vi "resonant.image queue to disk and to display queue_rrMD.vi"() -> ()   [LabVIEW 2012]
doc: "SciScan 1.0 151216"
uses:
  <vilib>/Utility/VariantDataType/Type.ctl
  Custom Controls/file format type def.ctl
  GFG/GFGnumericGet.vi
  GFG/GFGfpRefGet.vi
  GFG/GFGbooleanGet.vi
  image & display/save images/save channels to raw bin files.vi
  image & display/save images/save channels to interleaved multi-tiff files.vi
  image & display/save images/save channels to separate multi-tiff files.vi
  image & display/save images/save channels to stacked multi-tiff files.vi
  image & display/save images/save channels to interleaved tiff series.vi
  image & display/save images/save channels to separate tiff series.vi
  image & display/save images/save channels to stacked tiff series.vi
  GFG/GFG library.lvlib
  <vilib>/Utility/VariantDataType/VariantType.lvlib
panel:
  in  "Stop Button":bool
  out "VI is running":bool
  out "size(s)":i32[](array[numeric])
  out "error out 5":errorcluster
  out "error out 4":errorcluster
  out "error out 3":errorcluster
  out "error out 2":errorcluster
  out "# elements in image data queue":i32
  out "error out":errorcluster
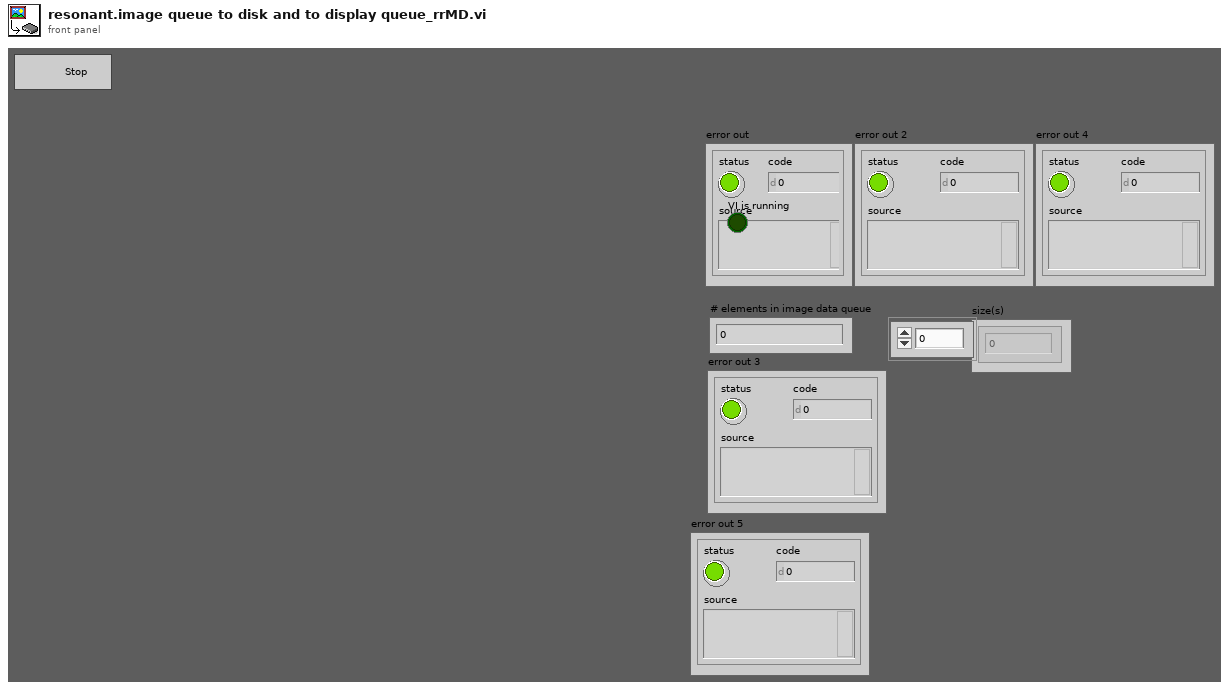
[diagram p1: front panel]
types:
  T1 = cluster{"Variable Name in":string, "Variant Out":variant}
  T2 = typedef "file format type def.ctl" = enum16{"16bit raw", "32bit raw", "16bit multi-tiff (interleave)", "16bit multi-tiff (separate)", "16bit multi-tiff (stacked)", "32bit multi-tiff (interleave)", "32bit multi-tiff (separate)", "32bit multi-tiff (stacked)", "16bit tiff series (interleave)", "16bit tiff series (separate)", "16bit tiff series (stacked)", "32bit tiff series (interleave)", "32bit tiff series (separate)", "32bit tiff series (stacked)"}
  T3 = enum8{"Enabled", "Disabled", "Disabled and Grayed Out"}
  T4 = cluster{"WaveformChartRef":refnum<vi>, "DigitalRef":refnum<vi>, "ArrayRef":refnum<vi>, "TabControlRef":refnum<vi>, "EnumRef":refnum<vi>, "RingRef":refnum<vi>, "BooleanRef":refnum<vi>, "KnobRef":refnum<vi>, "SlideRef":refnum<vi>, "PathRef":refnum<vi>, "StringRef":refnum<vi>, "ComboBox":refnum<vi>, "WaveformGraphRef":refnum<vi>}
  T5 = cluster{"NewVal":bool, "Event Registration Refnum":refnum<event-registration>}
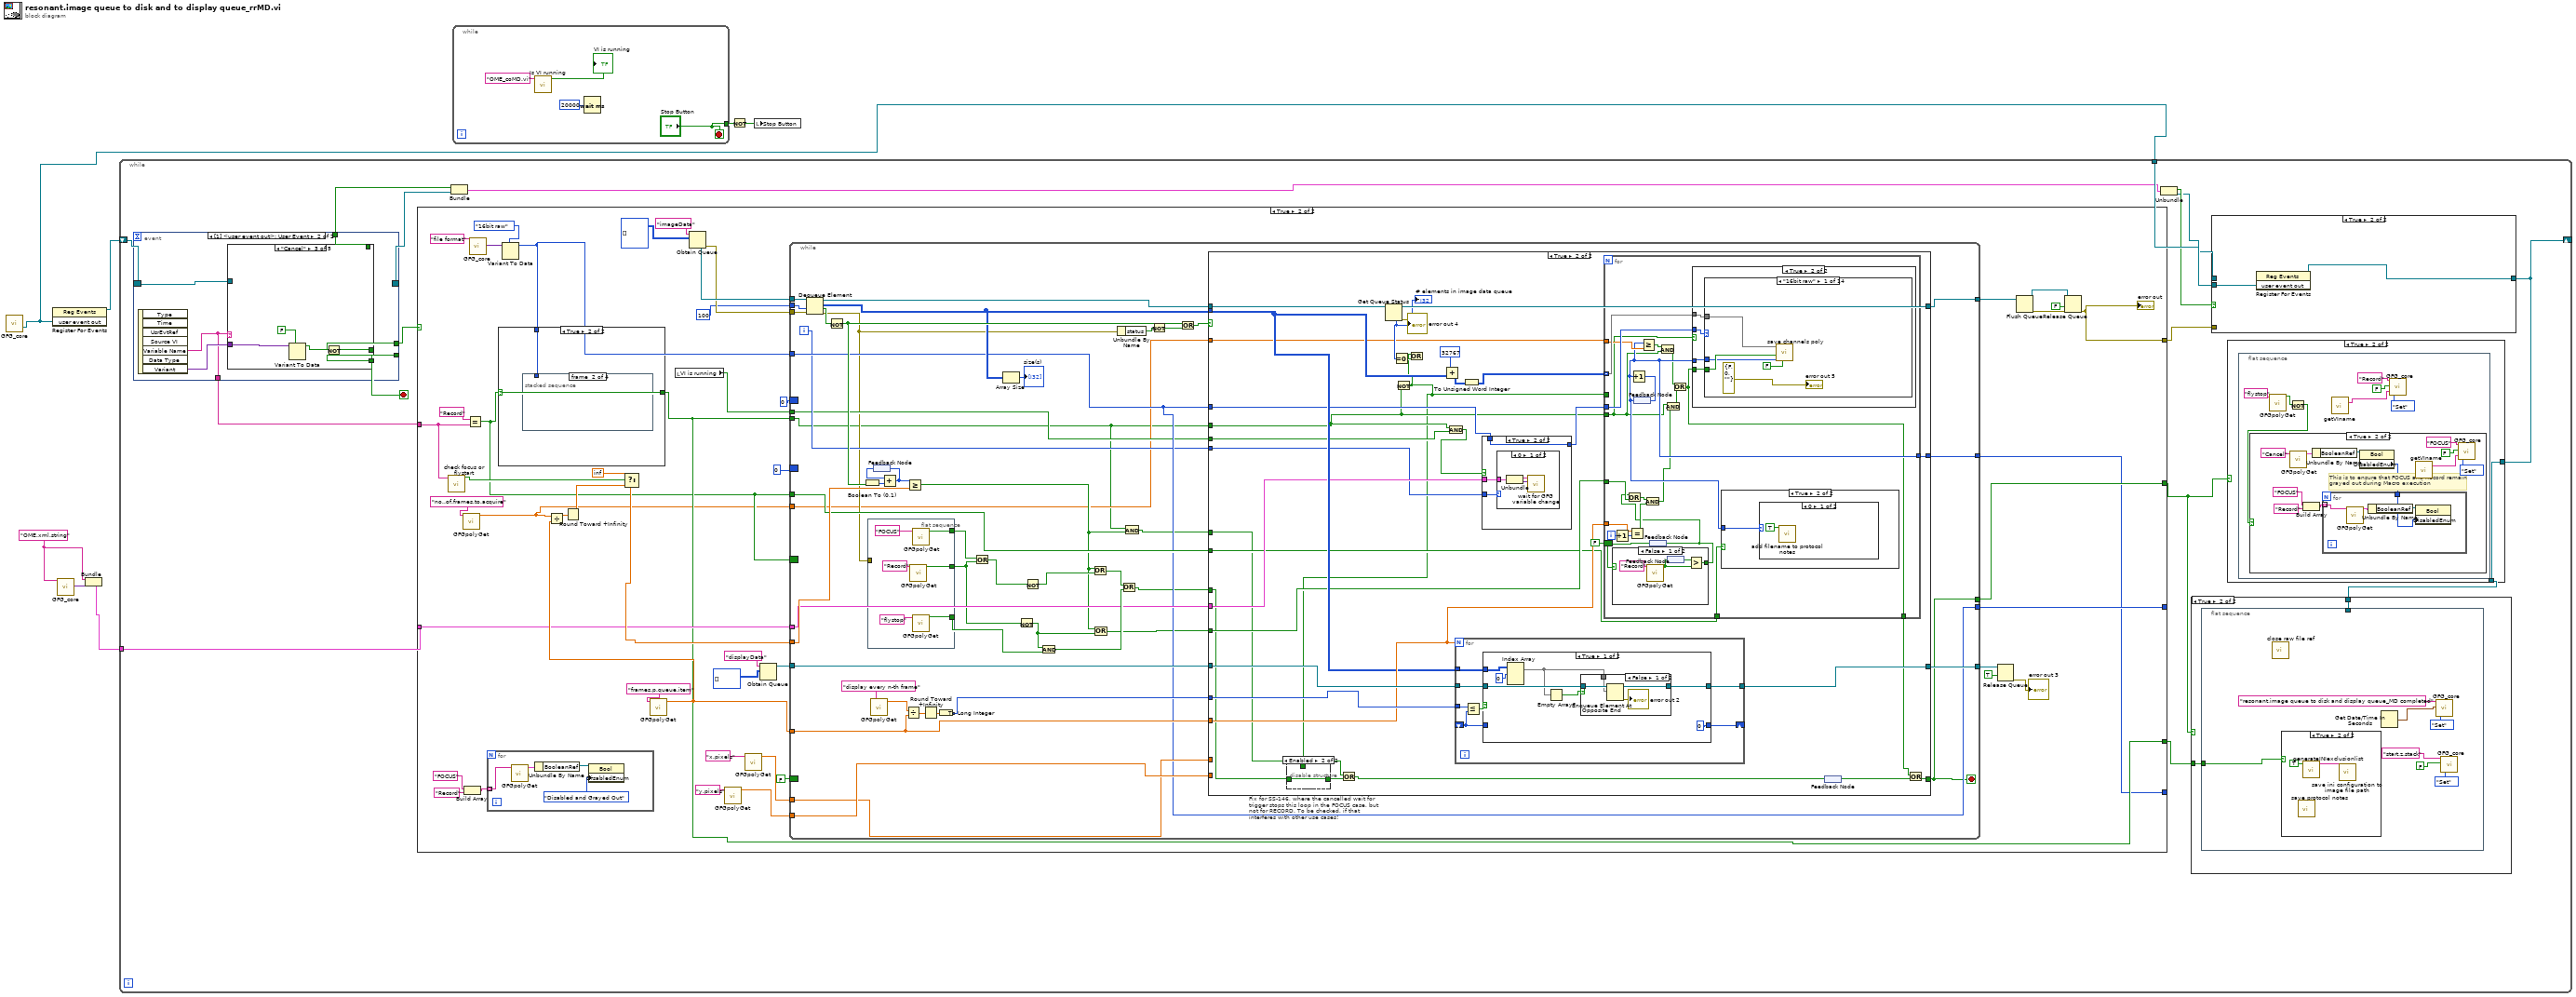
[diagram p0: block diagram]
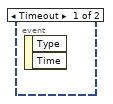
[diagram p7: hidden frame]
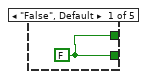
[diagram p8: hidden frame]
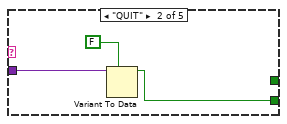
[diagram p9: hidden frame]
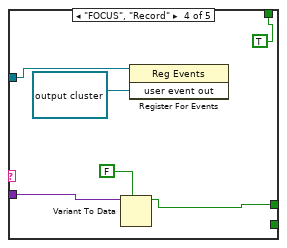
[diagram p10: hidden frame]
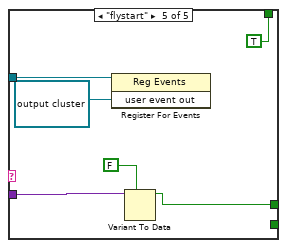
[diagram p11: hidden frame]
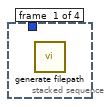
[diagram p14: hidden frame]
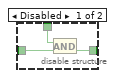
[diagram p18: hidden frame]
diagram:
  w4 = "OME.xml.string" ("Variable Name in")
  n1 = call "GFG_core.vi"() -> ("user event out"=w6:refnum<user-event>)  [unwired: 13 in, 6 out]
  n2 = register-events(w6) -> (reference out=w7:refnum<event-registration>)  [unwired: 2 in, 1 out]
  n3 = call "GFG_core.vi"("Variable Name in"=w4) -> ("Variant Out"=w5:variant)  [unwired: 12 in, 6 out]
  n4 = Bundle("Variable Name in"=w4, "Variant Out"=w5) -> (w3:T1)  [unwired: 1 in]
  n5 = while {
    shift-right: [w10] -> _
    shift-left: w7 -> [w20]
    tunnel: w6 -> [w19]
    tunnel: w3 -> [w12]
    stop <- w22 stop-if-true
    n6 = event shown="[1] <user event out>: User Event" {
      selector: w20 -> [_ w63]
      dyn-events: [_ _] -> w16
      timeout: _ -> [_ _]
      tunnel: [_ w67] -> w23
      tunnel: [_ w66] -> w22
      tunnel: [_ w64] -> w21
      tunnel: [_ w62] -> w17
      event Timeout {
        n7 = event-data() -> ()  [unwired: 1 in, 2 out]
      }
      event User Event {
        n8 = event-data() -> ("Variable Name"=w64:string, "Variant"=w65:variant)  [unwired: 1 in, 5 out]
        n9 = case shown="\"Cancel\"" w64 {
          tunnel: [w68 _ w72 w79 w85] -> w67
          tunnel: [w68 w69 _ _ _] -> w66
          tunnel: w65 -> [_ w71 w74 w80 w86]
          tunnel: w63 -> [_ _ _ w77 w83]
          tunnel: [_ _ _ TRUE ("NewVal") TRUE ("NewVal")] -> w62
          frame "False", Default {
            w68 = FALSE ("NewVal")
          }
          frame "QUIT" {
            n10 = Variant To Data(type=FALSE ("NewVal"), Variant=w71) -> (data=w69:bool)  [unwired: 1 in, 1 out]
          }
          frame "Cancel" {
            n11 = Variant To Data(type=FALSE ("NewVal"), Variant=w74) -> (data=w73:bool)  [unwired: 1 in, 1 out]
            n12 = Not(x=w73) -> (.not. x?=w72:bool)
          }
          frame "FOCUS", "Record" {
            n13 = Variant To Data(type=FALSE ("NewVal"), Variant=w80) -> (data=w79:bool)  [unwired: 1 in, 1 out]
            n14 = register-events(reference=w77, refnum<user-event> refnum ("user event out")) -> ()  [unwired: 1 in, 2 out]
          }
          frame "flystart" {
            n15 = register-events(reference=w83, refnum<user-event> refnum ("user event out")) -> ()  [unwired: 1 in, 2 out]
            n16 = Variant To Data(type=FALSE ("NewVal"), Variant=w86) -> (data=w85:bool)  [unwired: 1 in, 1 out]
          }
        }
      }
    }
    n17 = case shown="True" w23 {
      tunnel: w21 -> [_ w111]
      tunnel: [_ w120] -> w18
      tunnel: [_ w107] -> w8
      tunnel: w12 -> [_ w98]
      tunnel: [_ w97] -> w11
      tunnel: [_ w96] -> _
      tunnel: [_ w94] -> _
      frame False {
      }
      frame True {
        n18 = call "check focus or flystart.vi"("GFG variable name"=w111) -> ("Focus or flystart?"=w110:bool)  [unwired: 10 in]
        n19 = call-poly "GFGpolyGet.vi"("Variable Name in"="no..of.frames.to.acquire" ("Tag in")) -> ("Numeric"=w90:dbl)  [unwired: 8 in, 2 out]
        n20 = Build Array("FOCUS" ("Variable Name in"), "Record" ("element")) -> (w91:string[])
        n21 = Equal?(x="Record", y=w111) -> (x = y?=w95:bool)
        n22 = call "GFG_core.vi"("Variable Name in"="file format") -> ("Variant Out"=w125:variant)  [unwired: 12 in, 6 out]
        n23 = for {
          tunnel: w91 -> [w137] mode=indexing
          n24 = call-poly "GFGpolyGet.vi"("Variable Name in"=w137) -> ("output cluster"=w138:T4)  [unwired: 9 in, 1 out]
          n25 = Unbundle By Name(w138) -> ("BooleanRef"=w136:refnum<vi>)
          n26 = property class="Bool"(reference=w136, "DisabledEnum"=T3."Disabled and Grayed Out" ("Disabled")) -> ()  [unwired: 1 in, 2 out]
        }
        n27 = Variant To Data(type=file_format_type_def."16bit raw" ("file format"), Variant=w125) -> (data=w123:T2)  [unwired: 1 in, 1 out]
        n28 = case shown="True" w95 {
          selector: w95 -> [w140 w142]
          tunnel: [w140 w142] -> w97
          tunnel: w123 -> [_ w141]
          frame False {
          }
          frame True {
            n29 = stacked-sequence {
              tunnel: w141 -> [_ _ _ _]
              frame #0 {
                n30 = call "generate filepath.vi"() -> ()  [unwired: 11 in, 1 out]
              }
              frame #1 {
              }
              frame #2 {
              }
              frame #3 {
              }
            }
          }
        }
        n31 = call-poly "GFGpolyGet.vi"("Variable Name in"="frames.p.queue.item" ("Tag in")) -> ("Numeric"=w102:dbl)  [unwired: 8 in, 2 out]
        n32 = Divide(x=w90, y=w102) -> (x/y=w103:dbl)
        n33 = Round Toward +Infinity(x=w103) -> (ceil(x): smallest int >= x=w101:dbl)
        n34 = Select(t=inf, s=w110, f=w101) -> (s? t:f=w117:dbl)
        n35 = local read "VI is running"() -> (w88:bool)
        n36 = Obtain Queue(name (unnamed)="imageData", element data type=i16[][][] [] ("initialized array")) -> (queue out=w128:refnum<queue>, error out=w112:errorcluster)  [unwired: 3 in, 1 out]
        n37 = call-poly "GFGpolyGet.vi"("Variable Name in"="y.pixels" ("Tag in")) -> ("Numeric"=w114:dbl)  [unwired: 8 in, 2 out]
        n38 = call-poly "GFGpolyGet.vi"("Variable Name in"="x.pixels" ("Tag in")) -> ("Numeric"=w113:dbl)  [unwired: 8 in, 2 out]
        n39 = Obtain Queue(name (unnamed)="displayData", element data type=i16[][] [] ("initialized array")) -> (queue out=w134:refnum<queue>)  [unwired: 3 in, 2 out]
        n40 = while {
          tunnel: [w186] -> w132
          tunnel: w134 -> [w189]
          tunnel: [w190] -> w133
          tunnel: w117 -> [w164]
          tunnel: w128 -> [w188]
          tunnel: w97 -> [w145]
          tunnel: w123 -> [w159]
          tunnel: [w143] -> w107
          tunnel: w114 -> [w185]
          tunnel: w113 -> [w184]
          tunnel: w112 -> [w183]
          tunnel: 100 ("timeout in ms (-1)") -> [w181]
          tunnel: w102 -> [w179]
          border: 0 -> [_]
          border: i16 0 -> [_]
          tunnel: w95 -> [w163]
          tunnel: w98 -> [w160]
          tunnel: [w159] -> w96
          tunnel: w88 -> [w156]
          border: w95 -> [_]
          tunnel: [w150] -> w94
          tunnel: w90 -> [w147]
          border: FALSE -> [_]
          i -> [w158]
          stop <- w143 stop-if-true
          n41 = Dequeue Element(queue=w188, timeout in ms (-1)=w181, error in (no error)=w183) -> (queue out=w187:refnum<queue>, element=w162:i16[][][], timed out?=w182:bool, error out=w151:errorcluster)
          n42 = Not(x=w182) -> (.not. x?=w165:bool)
          n43 = Boolean To (0,1)(Boolean=w165) -> (0, 1=w168:i16)
          n44 = flat-sequence {
            tunnel: [w194] -> w177
            tunnel: [w192] -> w173
            tunnel: [w191] -> w154
            tunnel: w151 -> [_]
            frame #0 {
              n45 = call-poly "GFGpolyGet.vi"("Variable Name in"="Record") -> ("Boolean Value OUT"=w191:bool)  [unwired: 9 in, 1 out]
              n46 = call-poly "GFGpolyGet.vi"("Variable Name in"="flystop") -> ("Boolean Value OUT"=w192:bool)  [unwired: 9 in, 1 out]
              n47 = call-poly "GFGpolyGet.vi"("Variable Name in"="FOCUS") -> ("Boolean Value OUT"=w194:bool)  [unwired: 9 in, 1 out]
            }
          }
          n48 = call-poly "GFGpolyGet.vi"("Variable Name in"="display every n-th frame" ("Tag in")) -> ("Numeric"=w171:dbl)  [unwired: 8 in, 2 out]
          n49 = feedback #1() -> (w167:i16)
          n50 = Add(x=w167, y=w168) -> (x+y=w166:i16)
          n51 = feedback-in #1(w166) -> ()
          n52 = Divide(x=w171, y=w179) -> (x/y=w170:dbl)
          n53 = Greater Or Equal?(x=w166, y=w164) -> (x >= y?=w148:bool)
          n54 = Round Toward +Infinity(x=w170) -> (ceil(x): smallest int >= x=w169:dbl)
          n55 = To Long Integer(number=w169) -> (32bit integer=w180:i32)
          n56 = Or(x=w177, y=w154) -> (x .or. y?=w176:bool)
          n57 = Array Size(array=w162) -> (size(s)=→"size(s)":i32[])
          n58 = Not(x=w154) -> (.not. x?=w155:bool)
          n59 = Not(x=w176) -> (.not. x?=w175:bool)
          n60 = And(x=w155, y=w173) -> (x .and. y?=w178:bool)
          n61 = Or(x=w148, y=w175) -> (x .or. y?=w174:bool)
          n62 = Or(x=w148, y=w155) -> (x .or. y?=w157:bool)
          n63 = Unbundle By Name(w151) -> ("status"=w152:bool)
          n64 = Or(x=w174, y=w178) -> (x .or. y?=w153:bool)
          n65 = And(x=w145, y=w148) -> (x .and. y?=w146:bool)
          n66 = Not(x=w152) -> (.not. x?=w149:bool)
          n67 = Or(x=w165, y=w149) -> (x .or. y?=w161:bool)
          n68 = case shown="True" w161 {
            tunnel: [w198 w232] -> w190
            tunnel: w189 -> [w198 w231]
            tunnel: w187 -> [w199 w230]
            tunnel: [w199 w229] -> w186
            tunnel: w159 -> [_ w221]
            tunnel: w145 -> [_ w207]
            tunnel: w162 -> [_ w222]
            tunnel: w185 -> [_ _]
            tunnel: w184 -> [_ _]
            tunnel: w153 -> [w197 w216]
            tunnel: [w197 w206] -> w143
            tunnel: w180 -> [_ w227]
            tunnel: w179 -> [_ w224]
            tunnel: w163 -> [_ w215]
            tunnel: w160 -> [_ w220]
            tunnel: w158 -> [_ w219]
            tunnel: w157 -> [_ w217]
            tunnel: w156 -> [_ w208]
            tunnel: [_ w213] -> w150
            tunnel: w146 -> [_ w203]
            tunnel: w147 -> [_ w202]
            frame False {
            }
            frame True {
              n69 = Get Queue Status(queue=w230) -> (queue out=w229:refnum<queue>, error out=→"error out 4":errorcluster, # elements in queue=w212:i32)  [unwired: 2 in, 5 out]
              "# elements in image data queue" <- w212
              n70 = Equal To 0?(x=w212) -> (x = 0?=w210:bool)
              n71 = Not(x=w207) -> (.not. x?=w200:bool)
              n72 = disable-structure "Fix for SS-146, where the cancelled wait for trigger stops this loop in the FOCUS case, but not for RECORD. To be checked, if that interferes with other use cases!" shown="Enabled" {
                disable-tunnel: w216 -> [w235 w236]
                disable-tunnel: [w234 w236] -> w211
                disable-tunnel: w200 -> [w233 _]
                frame Disabled {
                  n73 = And(x=w233, y=w235) -> (x .and. y?=w234:bool)
                }
                frame Enabled {
                }
              }
              n74 = Or(x=w203, y=w211) -> (x .or. y?=w204:bool)
              n75 = Or(x=w200, y=w210) -> ()  [unwired: 1 out]
              n76 = Add(x=i16 32767, y=w222) -> (x+y=w226:i16[][][])
              n77 = And(x=w207, y=w208) -> (x .and. y?=w209:bool)
              n78 = for {
                N: w224 -> [_]
                tunnel: [w250] -> w232
                tunnel: w231 -> [w249]
                tunnel: w222 -> [w248]
                shift-right: [w247] -> _
                shift-left: _ -> [w244]
                tunnel: w227 -> [w246]
                n79 = Less Or Equal?(x=w246, y=w244) -> (x <= y?=w245:bool)
                n80 = case shown="True" w245 {
                  tunnel: [w257 w265] -> w250
                  tunnel: w249 -> [w256 w265]
                  tunnel: w248 -> [w254 _]
                  tunnel: [0 w263] -> w247
                  tunnel: w244 -> [_ w264]
                  frame True {
                    n81 = Index Array(array=w254, index (dim 0)=0 ("index (page)")) -> (element=w251:i16[][])  [unwired: 2 in]
                    n82 = Empty Array?(array=w251) -> (empty?=w255:bool)
                    n83 = case shown="False" w255 {
                      tunnel: [w261 w262] -> w257
                      tunnel: w256 -> [w260 w262]
                      tunnel: w251 -> [w258 _]
                      frame False {
                        n84 = Enqueue Element At Opposite End(queue=w260, element=w258) -> (queue out=w261:refnum<queue>, error out=→"error out 2":errorcluster)  [unwired: 2 in, 1 out]
                      }
                      frame True {
                      }
                    }
                  }
                  frame False {
                    n85 = Increment(x=w264) -> (x+1=w263:i32)
                  }
                }
              }
              n86 = To Unsigned Word Integer(number=w226) -> (unsigned 16bit integer=w228:u16[][][])
              n87 = case shown="True" w209 {
                tunnel: w221 -> [w237 w238]
                tunnel: w220 -> [_ w240]
                tunnel: w219 -> [_ w239]
                tunnel: [w237 w238] -> w218
                frame False {
                }
                frame True {
                  n88 = case shown="0" w239 {
                    tunnel: w240 -> [w243 _]
                    frame 0 {
                      n89 = Unbundle(w243) -> ("Variable Name in"=w242:string, "Variant Out"=w241:variant)
                      n90 = call "wait for GFG variable change.vi"("Initialization Value"=w241, "Variable Name in"=w242) -> ()  [unwired: 9 in, 1 out]
                    }
                    frame 1, Default {
                    }
                  }
                }
              }
              n91 = for {
                tunnel: w218 -> [w278]
                tunnel: w207 -> [w267]
                tunnel: w228 -> [w280] mode=indexing
                tunnel: w217 -> [w285]
                tunnel: w224 -> [w283]
                tunnel: w215 -> [w277]
                border: FALSE -> [_]
                tunnel: [w272] -> w213
                tunnel: w200 -> [_]
                tunnel: [w269] -> w205
                tunnel: w202 -> [w273]
                i -> [w284]
                n92 = Increment(x=w284) -> (x+1=w282:i32)
                n93 = Equal?(x=w283, y=w282) -> (x = y?=w279:bool)
                n94 = feedback #2() -> (w272:i32)
                n95 = Increment(x=w272) -> (x+1=w281:i32)
                n96 = feedback-in #2(w281) -> ()
                n97 = Greater Or Equal?(x=w272, y=w273) -> (x >= y?=w271:bool)
                n98 = feedback #3() -> (w276:bool)
                n99 = case shown="False" w276 {
                  selector: w276 -> [_ w290]
                  tunnel: [w286 w290] -> w274
                  frame False {
                    n100 = call-poly "GFGpolyGet.vi"("Variable Name in"="Record") -> ("Boolean Value OUT"=w288:bool)  [unwired: 9 in, 1 out]
                    n101 = feedback #4() -> (w287:bool)
                    n102 = feedback-in #4(w288) -> ()
                    n103 = Greater?(x=w287, y=w288) -> (0:w286:bool)
                  }
                  frame True {
                  }
                }
                n104 = Or(x=w274, y=w285) -> (x .or. y?=w275:bool)
                n105 = And(x=w275, y=w279) -> (x .and. y?=w266:bool)
                n106 = feedback-in #3(w274) -> ()
                n107 = And(x=w271, y=w267) -> (x .and. y?=w270:bool)
                n108 = And(x=w267, y=w266) -> (x .and. y?=w268:bool)
                n109 = Or(x=w270, y=w268) -> (x .or. y?=w269:bool)
                n110 = case shown="True" w267 {
                  tunnel: w269 -> [_ w295]
                  tunnel: w278 -> [_ w294]
                  tunnel: w280 -> [_ w296]
                  tunnel: w272 -> [_ w293]
                  frame False {
                  }
                  frame True {
                    n111 = case shown="\"16bit raw\"" w294 {
                      tunnel: w296 -> [w299 w303 w308 w311 w314 w317 w320 w323 w326 w329 w332 w335 w338 w341]
                      tunnel: w293 -> [w298 w305 w307 w310 w313 w316 w319 w322 w325 w328 w331 w334 w337 w340]
                      tunnel: w295 -> [w301 w304 w306 w309 w312 w315 w318 w321 w324 w327 w330 w333 w336 w339]
                      frame "16bit raw" {
                        n112 = call-poly "save channels poly.vi"("T:galvo F:resonant default:T"=FALSE, "frame number in"=w298, "last frame"=w301, "image data in (U16)"=w299) -> ()  [unwired: 8 in]
                        "error out 5" <- errorcluster {"status"=FALSE, "code"=0, "source"=""} ("error out 4")
                      }
                      frame "32bit raw" {
                        n113 = call-poly "save channels poly.vi"("T:galvo F:resonant default:T"=FALSE, "frame number in"=w305, "last frame"=w304, "image data in (SGL)"=w303) -> ()  [unwired: 8 in]
                      }
                      frame "16bit multi-tiff (interleave)" {
                        n114 = call-poly "save channels poly.vi"("frame number in"=w307, "last frame"=w306, "image data in"=w308) -> ()  [unwired: 9 in]
                      }
                      frame "16bit multi-tiff (separate)" {
                        n115 = call-poly "save channels poly.vi"("frame number in"=w310, "last frame"=w309, "image data in"=w311) -> ()  [unwired: 9 in]
                      }
                      frame "16bit multi-tiff (stacked)" {
                        n116 = call-poly "save channels poly.vi"("frame number in"=w313, "last frame"=w312, "image data in"=w314) -> ()  [unwired: 9 in]
                      }
                      frame "32bit multi-tiff (interleave)" {
                        n117 = call-poly "save channels poly.vi"("frame number in"=w316, "last frame"=w315, "image data in"=w317) -> ()  [unwired: 9 in]
                      }
                      frame "32bit multi-tiff (separate)" {
                        n118 = call-poly "save channels poly.vi"("frame number in"=w319, "last frame"=w318, "image data in"=w320) -> ()  [unwired: 9 in]
                      }
                      frame "32bit multi-tiff (stacked)" {
                        n119 = call-poly "save channels poly.vi"("frame number in"=w322, "last frame"=w321, "image data in"=w323) -> ()  [unwired: 9 in]
                      }
                      frame "16bit tiff series (interleave)" {
                        n120 = call-poly "save channels poly.vi"("frame number in"=w325, "last frame"=w324, "image data in"=w326) -> ()  [unwired: 9 in]
                      }
                      frame "16bit tiff series (separate)" {
                        n121 = call-poly "save channels poly.vi"("frame number in"=w328, "last frame"=w327, "image data in"=w329) -> ()  [unwired: 9 in]
                      }
                      frame "16bit tiff series (stacked)" {
                        n122 = call-poly "save channels poly.vi"("frame number in"=w331, "last frame"=w330, "image data in"=w332) -> ()  [unwired: 9 in]
                      }
                      frame "32bit tiff series (interleave)" {
                        n123 = call-poly "save channels poly.vi"("frame number in"=w334, "last frame"=w333, "image data in"=w335) -> ()  [unwired: 9 in]
                      }
                      frame "32bit tiff series (separate)" {
                        n124 = call-poly "save channels poly.vi"("frame number in"=w337, "last frame"=w336, "image data in"=w338) -> ()  [unwired: 9 in]
                      }
                      frame "32bit tiff series (stacked)" {
                        n125 = call-poly "save channels poly.vi"("frame number in"=w340, "last frame"=w339, "image data in"=w341) -> ()  [unwired: 9 in]
                      }
                    }
                  }
                }
                n126 = case shown="True" w277 {
                  tunnel: w272 -> [_ w291]
                  frame False {
                  }
                  frame True {
                    n127 = case shown="0" w291 {
                      frame 0 {
                        n128 = call "add filename to protocol notes.vi"("rec start/end (T is start)"=TRUE) -> ()  [unwired: 10 in, 1 out]
                      }
                      frame 1, Default {
                      }
                    }
                  }
                }
              }
              n129 = feedback-in #5(w204) -> ()
              n130 = feedback #5() -> (w201:bool)
              n131 = Or(x=w205, y=w201) -> (x .or. y?=w206:bool)
            }
          }
        }
        n132 = Release Queue(queue=w133, force destroy? (F)=TRUE) -> (error out=→"error out 3":errorcluster)  [unwired: 1 in, 2 out]
        n133 = Flush Queue(queue=w132) -> (queue out=w131:refnum<queue>, error out=w130:errorcluster)  [unwired: 1 in, 1 out]
        n134 = Release Queue(queue=w131, force destroy? (F)=FALSE, error in (no error)=w130) -> (error out=w120:errorcluster)  [unwired: 2 out]
        "error out" <- w120
      }
    }
    n135 = Bundle("NewVal"=w17, "Event Registration Refnum"=w16) -> (w15:T5)  [unwired: 1 in]
    n136 = Unbundle(w15) -> ("NewVal"=w14:bool, "Event Registration Refnum"=w13:refnum<event-registration>)
    n137 = case shown="True" w14 {
      tunnel: [w59 w61] -> w10
      tunnel: w19 -> [_ w60]
      tunnel: w18 -> [_ _]
      tunnel: w13 -> [w59 _]
      frame False {
      }
      frame True {
        n138 = register-events(w60) -> (reference out=w61:refnum<event-registration>)  [unwired: 2 in, 1 out]
      }
    }
    n139 = case shown="True" w8 {
      tunnel: [w35 w36] -> w9
      tunnel: w10 -> [w35 w36]
      frame False {
      }
      frame True {
        n140 = flat-sequence {
          frame #0 {
            n141 = call-poly "GFGpolyGet.vi"("Variable Name in"="flystop") -> ("Boolean Value OUT"=w43:bool)  [unwired: 9 in, 1 out]
            n142 = Not(x=w43) -> (.not. x?=w37:bool)
            n143 = case shown="True" w37 {
              frame False {
              }
              frame True {
                # "This is to ensure that FOCUS and Record remain\ngrayed out during Macro execution"
                n144 = call-poly "GFGpolyGet.vi"("Variable Name in"="Cancel") -> ("output cluster"=w46:T4)  [unwired: 9 in, 1 out]
                n145 = Build Array("FOCUS" ("Variable Name in"), "Record" ("element")) -> (w52:string[])
                n146 = Unbundle By Name(w46) -> ("BooleanRef"=w47:refnum<vi>)
                n147 = property class="Bool"(reference=w47) -> ("DisabledEnum"=w44:T3)  [unwired: 1 in, 2 out]
                n148 = for {
                  tunnel: w52 -> [w57] mode=indexing
                  tunnel: w44 -> [w55]
                  n149 = call-poly "GFGpolyGet.vi"("Variable Name in"=w57) -> ("output cluster"=w58:T4)  [unwired: 9 in, 1 out]
                  n150 = Unbundle By Name(w58) -> ("BooleanRef"=w56:refnum<vi>)
                  n151 = property class="Bool"(reference=w56, "DisabledEnum"=w55) -> ()  [unwired: 1 in, 2 out]
                }
                n152 = call "getVIname.vi"() -> ("VI name"=w51:string)  [unwired: 19 in]
                n153 = call "GFG_core.vi"("Variable Name in"="FOCUS" ("Tag in"), "Variant in"=FALSE, "Source VI"=w51, "Action"=enum16{"Init", "Set", "Get"}."Set") -> ()  [unwired: 9 in, 7 out]
              }
            }
            n154 = call "getVIname.vi"() -> ("VI name"=w38:string)  [unwired: 19 in]
            n155 = call "GFG_core.vi"("Variable Name in"="Record" ("Tag in"), "Variant in"=FALSE, "Source VI"=w38, "Action"=enum16{"Init", "Set", "Get"}."Set") -> ()  [unwired: 9 in, 7 out]
          }
        }
      }
    }
    n156 = case shown="True" w8 {
      tunnel: w11 -> [_ w25]
      tunnel: w9 -> [_ w24]
      frame False {
      }
      frame True {
        n157 = flat-sequence {
          tunnel: w24 -> [_]
          tunnel: w25 -> [w29]
          frame #0 {
            n158 = call "close raw file ref.vi"() -> ()  [unwired: 12 in]
            n159 = case shown="True" w29 {
              frame False {
              }
              frame True {
                n160 = call "save protocol notes.vi"() -> ()  [unwired: 12 in]
                n161 = call "generateINIexclusionlist.vi"("T for reso, F for galvo"=TRUE) -> ("Array"=w34:string[])  [unwired: 10 in]
                n162 = call "save ini configuration to image file path.vi"("exclusion regexp array"=w34) -> ()  [unwired: 11 in]
              }
            }
            n163 = Get Date/Time In Seconds() -> (seconds since 1Jan1904=w30:timestamp)
            n164 = call "GFG_core.vi"("Variable Name in"="resonant.image queue to disk and display queue_MD completed", "Variant in"=w30, "Action"=enum16{"Init", "Set", "Get"}."Set") -> ()  [unwired: 10 in, 7 out]
            n165 = call "GFG_core.vi"("Variable Name in"="start.z.stack", "Variant in"=FALSE ("T for grey out"), "Action"=enum16{"Init", "Set", "Get"}."Set") -> ()  [unwired: 10 in, 7 out]
          }
        }
      }
    }
  }
  n166 = while {
    tunnel: ["Stop Button"] -> w2
    stop <- "Stop Button" stop-if-true
    n167 = call "Is VI running.vi"("VI name"="OME_coMD.vi") -> ("VI is running"=→"VI is running":bool)  [unwired: 9 in, 1 out]
    n168 = Wait (ms)(milliseconds to wait=u32 20000) -> ()  [unwired: 1 out]
  }
  n169 = Not(x=w2) -> (.not. x?=w1:bool)
  n170 = local write "Stop Button"(w1) -> ()
